vi "Read.vi"(8 "error in (no error)":errorcluster caption="entrée d'erreur (pas d'erreur)", 11 "Class DIO (Default) en entrée":refnum<class "Class Ana NI.lvclass">) -> (0 "error out":errorcluster caption="sortie d'erreur", 3 "Class DIO (Default) en sortie":refnum<class "Class Ana NI.lvclass">)   [LabVIEW 2020, in "Library Instrument & Equipement.lvlib" / "Library Ana.lvlib" / "Class Ana NI.lvclass"]
uses:
  Class Ana NI.lvclass
  C:/Users/ngarcin/OneDrive - Altyor/Standard TB/Class/Ana/Class Ana (Default)/Class Ana (Default).lvclass
  <vilib>/DAQmx/read.llb/DAQmx Read (Analog 1D Wfm NChan NSamp).vi
  <vilib>/DAQmx/miscellaneous.llb/DAQmx Fill In Error Info.vi
  Class Ana NI.lvclass/Class Ana NI.ctl
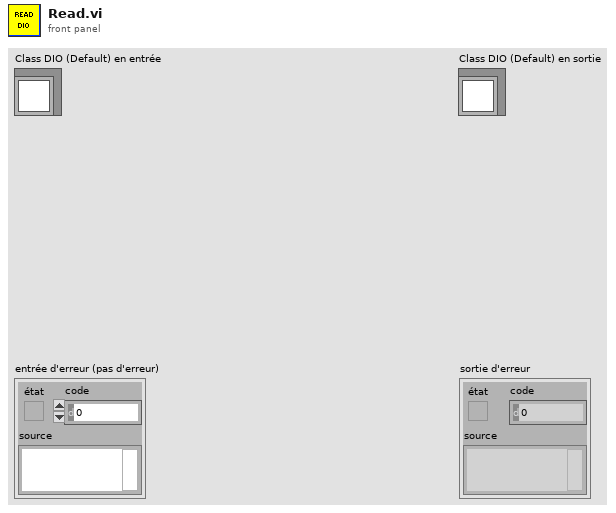
[diagram p1: front panel]
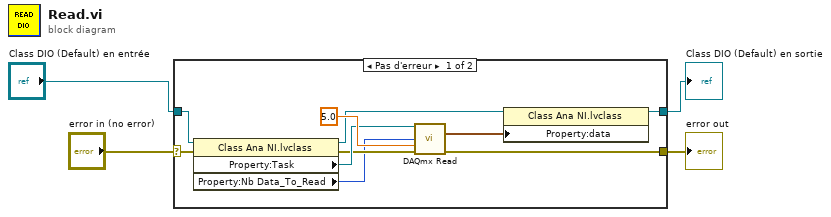
[diagram p0: block diagram]
diagram:
  n1 = case shown="Pas d'erreur" "error in (no error)" {
    selector: "error in (no error)" -> [w13 w16]
    tunnel: [w9 w16] -> w3
    tunnel: [w6 w15] -> w1
    tunnel: "Class DIO (Default) en entrée" -> [w14 w15]
    frame No Error {
      n2 = property class="Class Ana NI.lvclass"(reference=w14, error in=w13) -> (reference out=w7:refnum<class "Class Ana NI.lvclass">, error out=w10:errorcluster, "Property:Task"=w11:refnum<k21>, "Property:Nb Data_To_Read"=w5:i16)
      n3 = call-poly <vilib>:"DAQmx Read.vi"("task/channels in"=w11, "number of samples per channel"=w5, "timeout"=5.0, "error in"=w10) -> ("data"=w8:waveform(dbl)[], "error out"=w9:errorcluster)  [unwired: 9 in, 1 out]
      n4 = property class="Class Ana NI.lvclass"(reference=w7, "Property:data"=w8) -> (reference out=w6:refnum<class "Class Ana NI.lvclass">)  [unwired: 1 in, 1 out]
    }
    frame Error {
    }
  }
  "error out" <- w3
  "Class DIO (Default) en sortie" <- w1
